vi "StringToModeEnum.vi"(3 "Input String":string) -> (7 "Output Enum":T1)   [LabVIEW 2024]
uses:
  <userlib>/_OpenG.lib/lvdata/lvdata.llb/openg_variant.lvlib
  DataTypes/Mode.ctl
panel:
  in  "Input Enum":T1
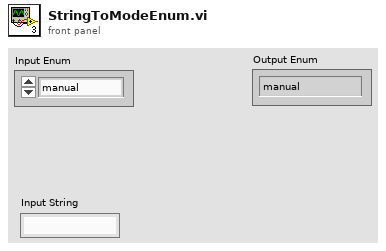
[diagram p1: front panel]
types:
  T1 = typedef "Mode.ctl" = enum16{"manual", "auto"}
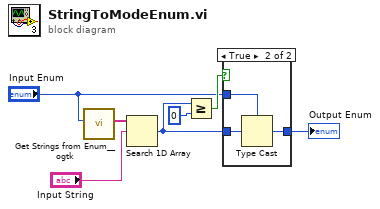
[diagram p0: block diagram]
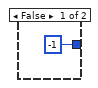
[diagram p2: hidden frame]
diagram:
  n1 = call <userlib>:"Get Strings from Enum__ogtk.vi"("Enum"="Input Enum") -> ("Enum Strings"=w7:string[])  [unwired: 7 in, 3 out]
  n2 = Search 1D Array(1D array=w7, element="Input String") -> (index of element=w3:i32)  [unwired: 1 in]
  n3 = Greater Or Equal?(x=w3, y=0) -> (x >= y?=w5:bool)
  n4 = case shown="True" w5 {
    tunnel: w3 -> [_ w11]
    tunnel: [-1 w9] -> w1
    tunnel: "Input Enum" -> [_ w10]
    frame False {
    }
    frame True {
      n5 = Type Cast(type=w10, x=w11) -> (*(type *) &x=w9:T1)
    }
  }
  "Output Enum" <- w1
